vi "Enumerated Windows_KT.vi"() -> (1 "Windows":string[](array[string]), 3 "hWnd":u32[](array[numeric]))   [LabVIEW 2017, in "KTools.lvlib"]
doc: "<-------Enumerated Windows------->\nEnumerates all the top level window handles and names."
uses:
  KTools.lvlib
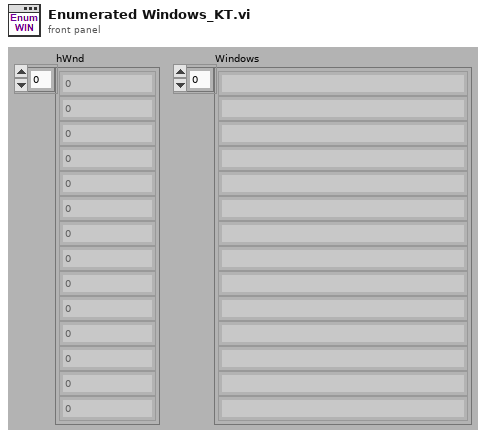
[diagram p1: front panel]
types:
  T1 = enum8{"First", "Last", "Next", "Previous", "Owner", "Child"}
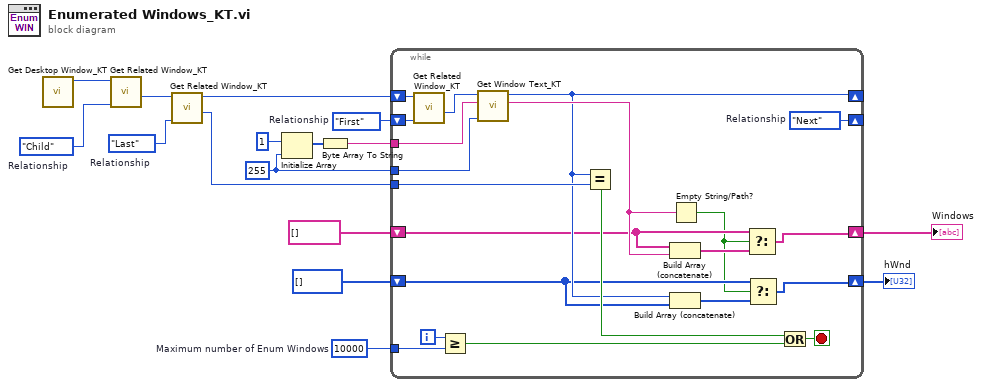
[diagram p0: block diagram]
diagram:
  w1 = T1."First"  # Relationship
  w2 = T1."Last"  # Relationship
  w3 = T1."Child"  # Relationship
  w5 = 10000  # Maximum number of Enum Windows
  w15 = 255 ("dimension size")
  n1 = call "Get Desktop Window_KT.vi"() -> ("hWnd"=w4:u32)  [unwired: 9 in]
  n2 = call "Get Related Window_KT.vi"("Relationship"=w3, "hWnd"=w4) -> ("hWnd related"=w9:u32)  [unwired: 6 in, 1 out]
  n3 = call "Get Related Window_KT.vi"("Relationship"=w2, "hWnd"=w9) -> ("hWnd related"=w10:u32, "hWnd dup"=w8:u32)  [unwired: 6 in]
  n4 = Initialize Array(1 ("uCmd"), w15) -> (w13:i32[])
  n5 = Byte Array To String(unsigned byte array=w13) -> (string=w14:string)
  n6 = while {
    tunnel: w15 -> [w29]
    tunnel: w14 -> [w28]
    tunnel: w10 -> [w37]
    shift-right: [w17] -> w7
    shift-left: u32[] [] ("hWnd") -> [w19]
    shift-right: [w21] -> w11
    shift-left: string[] [] ("Windows") -> [w23]
    shift-right: [w24] -> _
    shift-left: w1 -> [w35]
    shift-right: [w26] -> _
    shift-left: w8 -> [w36]
    tunnel: w5 -> [w33]
    i -> [w34]
    stop <- w30 stop-if-true
    w24 = T1."Next"  # Relationship
    n7 = call "Get Related Window_KT.vi"("Relationship"=w35, "hWnd"=w36) -> ("hWnd related"=w25:u32)  [unwired: 6 in, 1 out]
    n8 = Greater Or Equal?(x=w34, y=w33) -> (x >= y?=w32:bool)
    n9 = call "Get Window Text_KT.vi"("nMaxCount"=w29, "Name (Byte)"=w28, "hWnd"=w25) -> ("Name"=w27:string, "hWnd dup"=w26:u32)  [unwired: 5 in]
    n10 = Equal?(x=w26, y=w37) -> (x = y?=w31:bool)
    n11 = Build Array (concatenate)(w23, w27) -> (w22:string[])
    n12 = Build Array (concatenate)(w26, w19) -> (w20:u32[])
    n13 = Empty String/Path?(string/path=w27) -> (empty?=w18:bool)
    n14 = Select(t=w23, s=w18, f=w22) -> (s? t:f=w21:string[])
    n15 = Select(t=w19, s=w18, f=w20) -> (s? t:f=w17:u32[])
    n16 = Or(x=w31, y=w32) -> (x .or. y?=w30:bool)
  }
  "Windows" <- w11
  "hWnd" <- w7
